vi "Wait.vi"(8 "error in (no error)":errorcluster, 11 "Serial in":refnum<class "Serial.lvclass">) -> (0 "error out":errorcluster, 2 "Ready?":bool, 3 "Serial out":refnum<class "Serial.lvclass">)   [LabVIEW 2021, in "Serial.lvclass"]
uses:
  Serial.lvclass
  Serial.lvclass/Serial.ctl
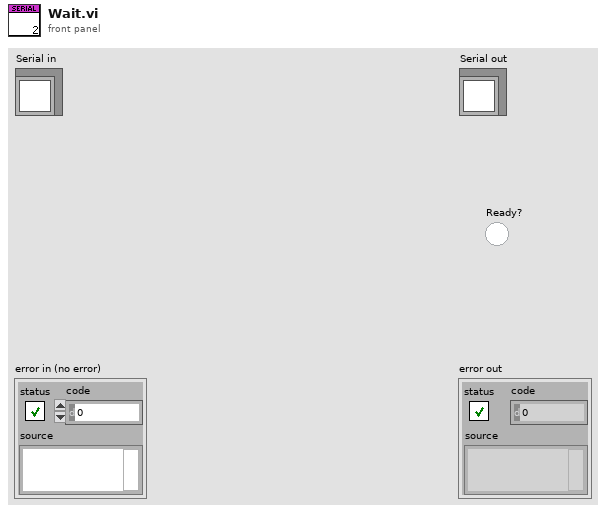
[diagram p1: front panel]
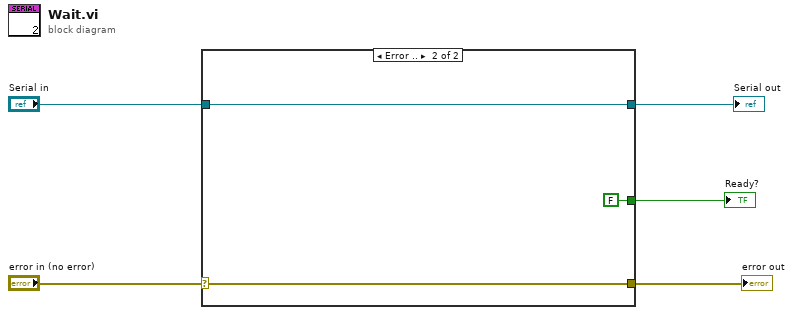
[diagram p0: block diagram]
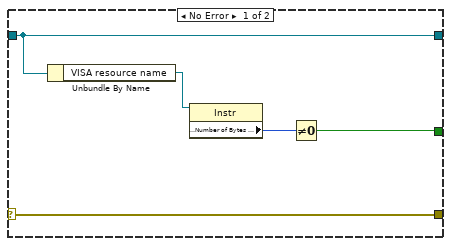
[diagram p2: hidden frame]
diagram:
  n1 = case shown="Error .." "error in (no error)" {
    selector: "error in (no error)" -> [w8 w13]
    tunnel: "Serial in" -> [w9 w12]
    tunnel: [w9 w12] -> w3
    tunnel: [w8 w13] -> w2
    tunnel: [w6 FALSE] -> w1
    frame No Error {
      n2 = Unbundle By Name(w9) -> ("VISA resource name"=w10:refnum<visa-resource-name>)
      n3 = property class="Instr"(reference=w10) -> ("Serial Settings:Number of Bytes at Serial Port"=w7:u32)  [unwired: 1 in, 2 out]
      n4 = Not Equal To 0?(x=w7) -> (x != 0?=w6:bool)
    }
    frame Error {
    }
  }
  "error out" <- w2
  "Serial out" <- w3
  "Ready?" <- w1
